vi "Assign Pixel to Wing Sector (FPGA).vi"(4 "End of Data?":bool, 6 "Valid Data?":bool, 7 "Pixel Intensity In":u8, 8 "Right Wing?":bool, 9 "Sector Parameters":T1, 10 "Pixel Y":u16, 11 "Pixel X":u16) -> (0 "Y Pixel Out":u16, 1 "Pixel Intensity Out":u8, 2 "sector #":u8, 3 "output valid":bool, 5 "X Pixel Out":u16)   [LabVIEW 2013]
uses:
  Sector Parameter Cluster.ctl
  <vilib>/rvi/FXPMathLib/FxpRectToPolar/XNode/nifxpmath_RectToPolar.xnode
  <vilib>/rvi/FXPMathLib/FxpSub/XNode/nifxpmath_Sub.xnode
  <vilib>/rvi/FXPMathLib/sim/FxpSim.dll
  <vilib>/rvi/FXPMathLib/FxpAdd/XNode/nifxpmath_Add.xnode
  <vilib>/rvi/FXPMathLib/FxpDiv/XNode/nifxpmath_Div.xnode
  <vilib>/rvi/FXPMathLib/FxpRectToPolar/simVIs/DllFxpRectToPolarTemp_sub.vi
  <vilib>/rvi/FXPMathLib/FxpRectToPolar/subVIs/nifxpmath_RectToPolar_SimConfig.ctl
  <vilib>/ptbypt/NI_PtbyPt.lvlib
  <vilib>/rvi/FXPMathLib/FxpDiv/simVIs/DllFxpDivTemp_sub.vi
  <vilib>/rvi/FXPMathLib/FxpDiv/subVIs/nifxpmath_Div_SimConfig.ctl
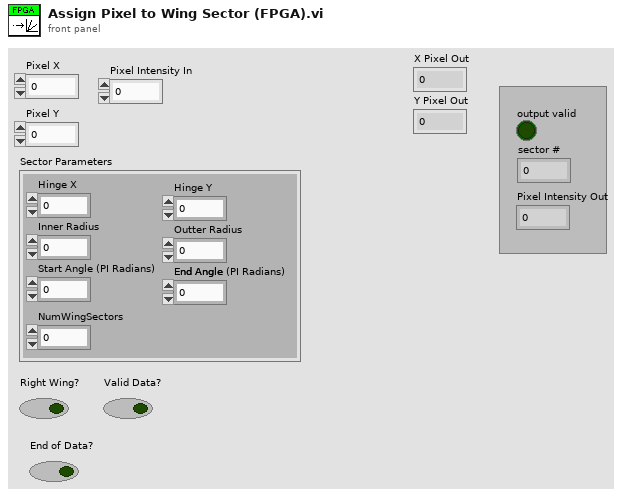
[diagram p1: front panel]
types:
  T1 = typedef "Sector Parameter Cluster.ctl" = cluster{"Start Angle":fxp<+/-,17,2>, "End Angle":fxp<+/-,17,2>, "Inner Radius":u16, "Outter Radius":u16, "Hinge X":u16, "Hinge Y":u16, "NumWingSectors":u8}
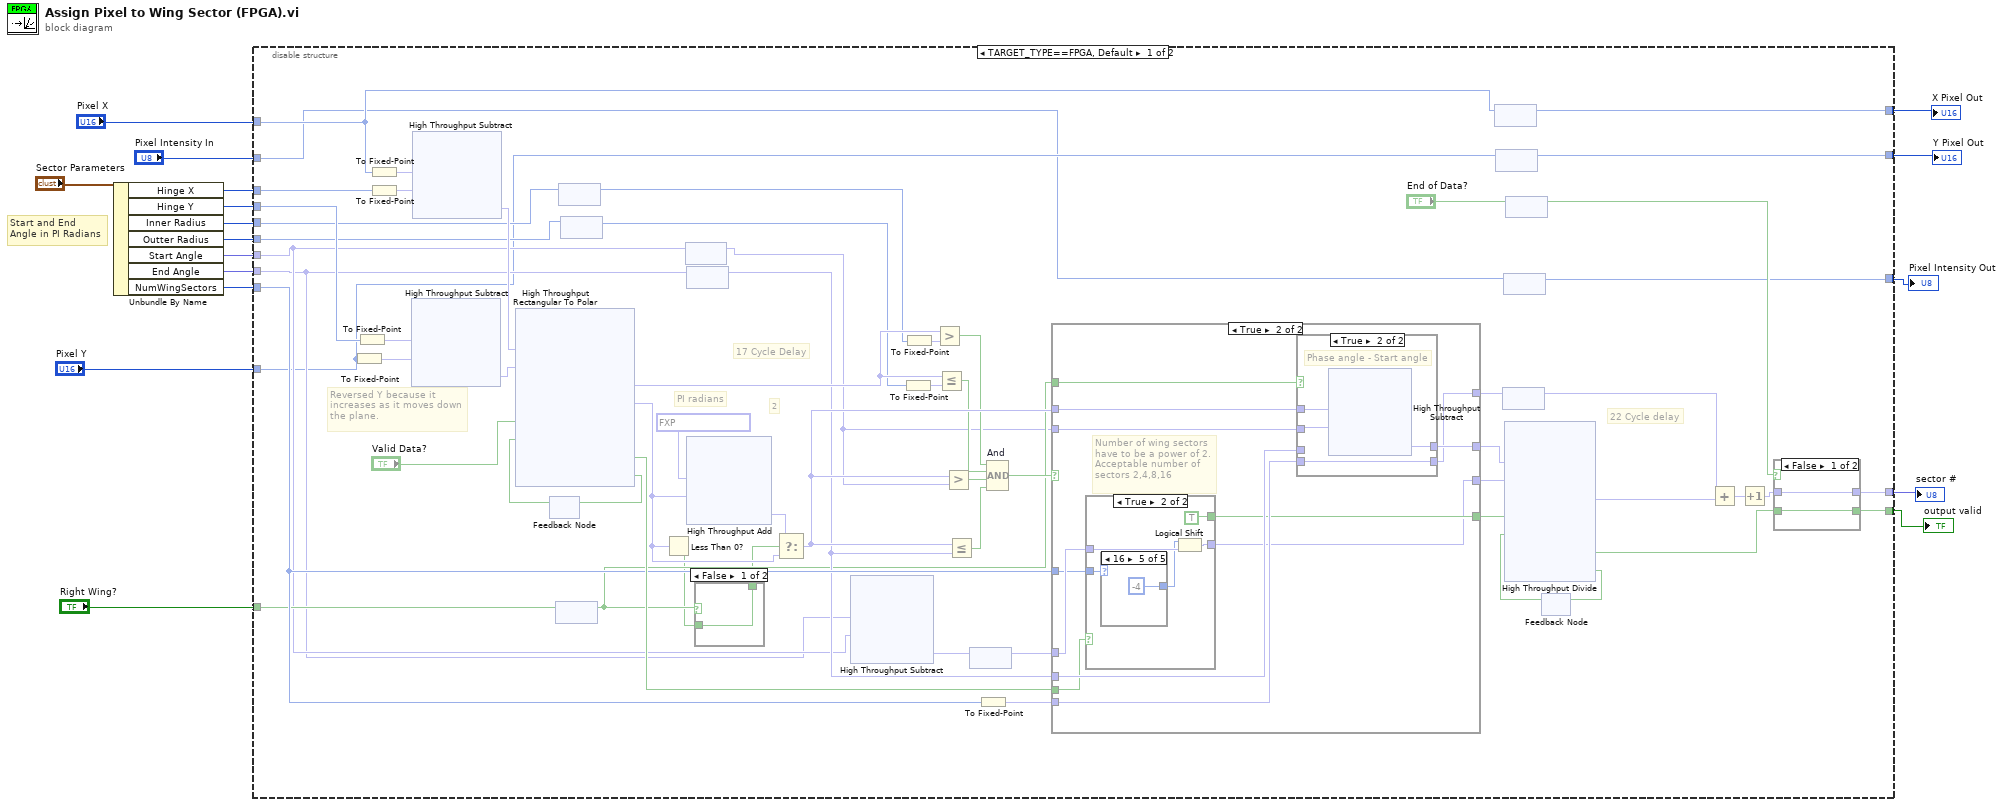
[diagram p0: block diagram]
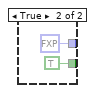
[diagram p2: hidden frame]
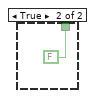
[diagram p3: hidden frame]
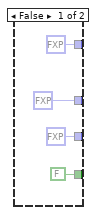
[diagram p4: hidden frame]
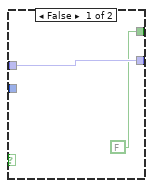
[diagram p5: hidden frame]
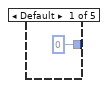
[diagram p6: hidden frame]
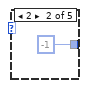
[diagram p7: hidden frame]
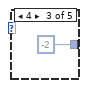
[diagram p8: hidden frame]
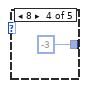
[diagram p9: hidden frame]
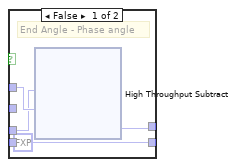
[diagram p10: hidden frame]
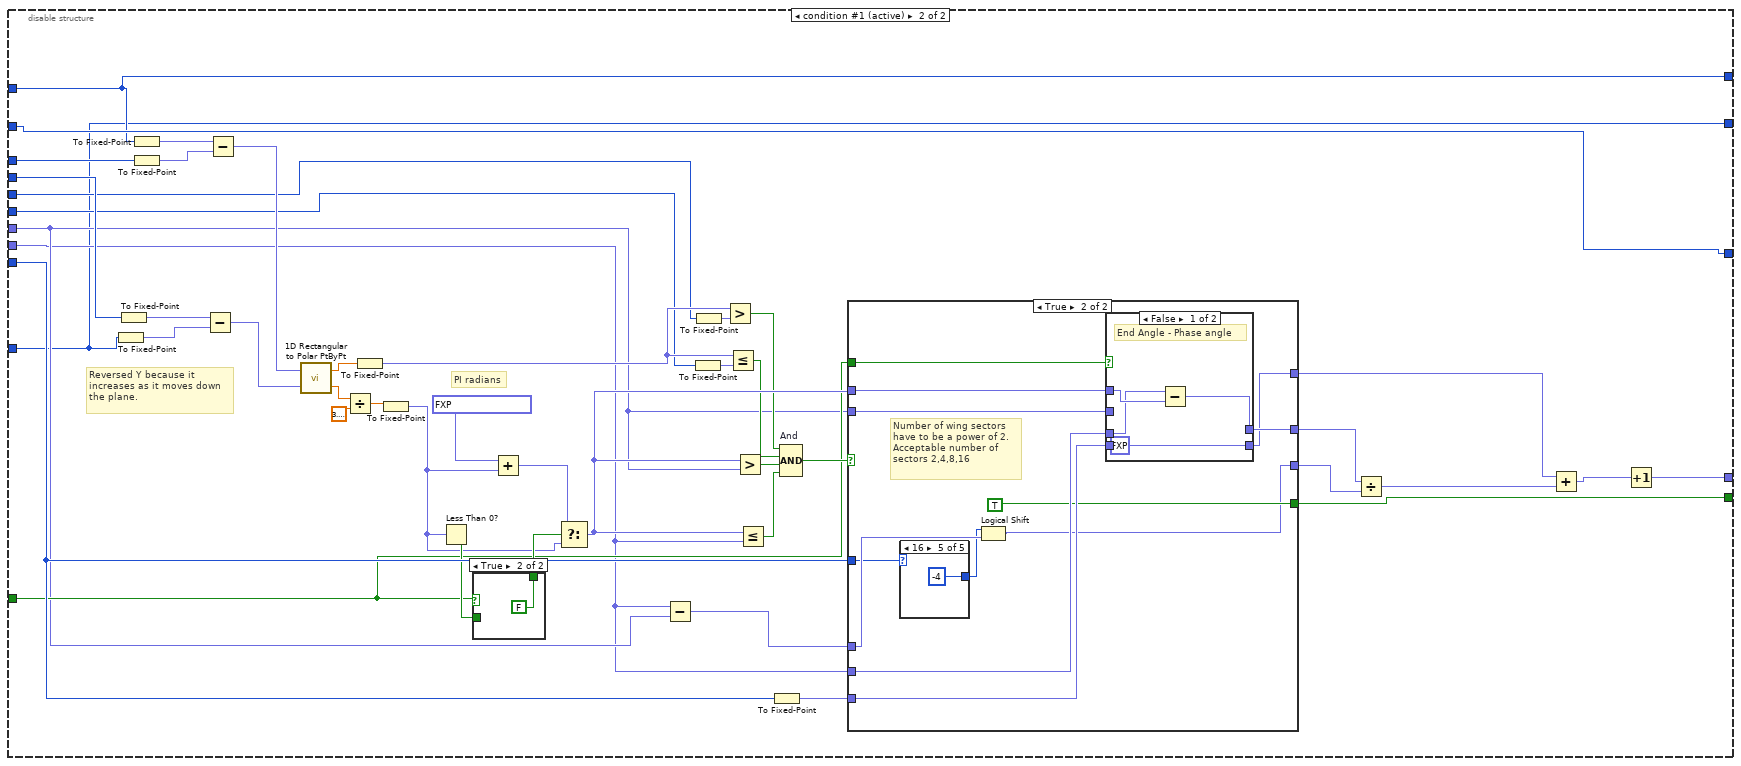
[diagram p11: hidden frame]
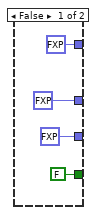
[diagram p13: hidden frame]
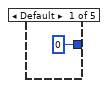
[diagram p14: hidden frame]
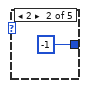
[diagram p15: hidden frame]
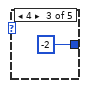
[diagram p16: hidden frame]
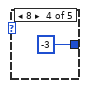
[diagram p17: hidden frame]
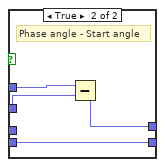
[diagram p18: hidden frame]
diagram:
  # "Start and End\nAngle in PI Radians"
  n1 = Unbundle By Name("Sector Parameters") -> ("Hinge X"=w15:u16, "Hinge Y"=w17:u16, "Inner Radius"=w13:u16, "Outter Radius"=w12:u16, "Start Angle"=w10:fxp<+/-,17,2>, "End Angle"=w9:fxp<+/-,17,2>, "NumWingSectors"=w16:u8)
  n2 = disable-structure shown="TARGET_TYPE==FPGA, Default" {
    disable-tunnel: w17 -> [w64 w222]
    disable-tunnel: w16 -> [w50 w214]
    disable-tunnel: w15 -> [w49 w213]
    disable-tunnel: w13 -> [w48 w202]
    disable-tunnel: w12 -> [w46 w201]
    disable-tunnel: "Right Wing?" -> [w40 w203]
    disable-tunnel: w10 -> [w37 w200]
    disable-tunnel: w9 -> [w35 w199]
    disable-tunnel: [w29 w190] -> w8
    disable-tunnel: [w27 w194] -> w7
    disable-tunnel: "Pixel X" -> [w25 w196]
    disable-tunnel: "Pixel Y" -> [w24 w195]
    disable-tunnel: [w23 w196] -> w4
    disable-tunnel: [w22 w195] -> w3
    disable-tunnel: [w21 w197] -> w2
    disable-tunnel: "Pixel Intensity In" -> [w20 w197]
    frame condition #0 {
      # "17 Cycle Delay"
      # "Reversed Y because it\nincreases as it moves down\nthe plane."
      # "PI radians"
      # "22 Cycle delay"
      # "2"
      n3 = To Fixed-Point(number=w24) -> (fixed-point=w54:fxp<+,11,11>)  [unwired: 1 in]
      n4 = To Fixed-Point(number=w64) -> (fixed-point=w55:fxp<+,11,11>)  [unwired: 1 in]
      n5 = To Fixed-Point(number=w25) -> (fixed-point=w53:fxp<+,11,11>)  [unwired: 1 in]
      n6 = To Fixed-Point(number=w49) -> (fixed-point=w52:fxp<+,11,11>)  [unwired: 1 in]
      n7 = xnode "High Throughput Subtract"("x"=w55, "y"=w54) -> ("x-y"=w63:fxp<+/-,12,12>)
      n8 = xnode "High Throughput Subtract"("x"=w53, "y"=w52) -> ("x-y"=w62:fxp<+/-,12,12>)
      n9 = feedback #1() -> (w69:bool)  [unwired: 1 in]
      n10 = xnode "High Throughput Rectangular To Polar"("x"=w62, "y"=w63, "input valid"="Valid Data?", "ready for output (T)"=w69) -> ("magnitude"=w77:fxp<+,12,12>, "phase (pi)"=w74:fxp<+/-,16,2>, "output valid"=w51:bool, "ready for input"=w70:bool)
      n11 = feedback-in #1(w70) -> ()
      n12 = feedback #2() -> (w43:bool)  [unwired: 1 in]
      n13 = feedback-in #2(w40) -> ()
      n14 = feedback #3() -> (w47:u16)  [unwired: 1 in]
      n15 = feedback-in #3(w48) -> ()
      n16 = feedback #4() -> (w45:u16)  [unwired: 1 in]
      n17 = feedback-in #4(w46) -> ()
      n18 = Less Than 0?(x=w74) -> (x < 0?=w41:bool)
      n19 = feedback #5() -> (w36:fxp<+/-,17,2>)  [unwired: 1 in]
      n20 = feedback-in #5(w37) -> ()
      n21 = xnode ("High Throughput Add")("x"=fxp<+/-,16,2> 1.99993896484375 ("y"), "y"=w74) -> ("x+y"=w73:fxp<+/-,17,3>)
      n22 = feedback #6() -> (w44:fxp<+/-,17,2>)  [unwired: 1 in]
      n23 = feedback-in #6(w35) -> ()
      n24 = case shown="False" w43 {
        tunnel: [w83 FALSE ("s")] -> w42
        tunnel: w41 -> [w83 _]
        frame False {
        }
        frame True {
        }
      }
      n25 = Select(t=w73, s=w42, f=w74) -> (s? t:f=w71:fxp<+/-,17,3>)
      n26 = xnode ("High Throughput Subtract")("x"=w35, "y"=w37) -> ("x-y"=w34:fxp<+/-,18,3>)
      n27 = To Fixed-Point(number=w45) -> (fixed-point=w76:fxp<+,16,16>)  [unwired: 1 in]
      n28 = To Fixed-Point(number=w47) -> (fixed-point=w78:fxp<+,16,16>)  [unwired: 1 in]
      n29 = Greater?(x=w77, y=w78) -> (0:w68:bool)
      n30 = Less Or Equal?(x=w77, y=w76) -> (x <= y?=w67:bool)
      n31 = Greater?(x=w71, y=w36) -> (0:w66:bool)
      n32 = Less Or Equal?(x=w71, y=w44) -> (x <= y?=w65:bool)
      n33 = feedback #7() -> (w33:fxp<+/-,18,3>)  [unwired: 1 in]
      n34 = feedback-in #7(w34) -> ()
      n35 = To Fixed-Point(number=w50) -> (fixed-point=w39:fxp<+,8,8>)  [unwired: 1 in]
      n36 = Compound Arithmetic op=AND "And"(w68, w67, w66, w65) -> (w75:bool)
      n37 = case shown="True" w75 {
        tunnel: w71 -> [_ w129]
        tunnel: w36 -> [_ w128]
        tunnel: [fxp<+/-,18,3> 0.0 ("x-y") w119] -> w59
        tunnel: w44 -> [_ w126]
        tunnel: w39 -> [_ w127]
        tunnel: [fxp<+/-,20,5> 0.0 ("x-y") w125] -> w60
        tunnel: [FALSE ("output valid") w120] -> w58
        tunnel: [fxp<+,8,8> 0.0 w124] -> w56
        tunnel: w33 -> [_ w123]
        tunnel: w51 -> [_ w122]
        tunnel: w50 -> [_ w121]
        tunnel: w43 -> [_ w118]
        frame False {
        }
        frame True {
          # "Number of wing sectors\nhave to be a power of 2.\nAcceptable number of\nsectors 2,4,8,16"
          n38 = case shown="True" w122 {
            tunnel: w121 -> [_ w136]
            tunnel: w123 -> [w131 w135]
            tunnel: [w131 w133] -> w119
            tunnel: [FALSE ("output valid") TRUE ("output valid")] -> w120
            frame False {
            }
            frame True {
              n39 = case shown="16" w136 {
                tunnel: [i16 0 ("y") i16 -1 ("y") i16 -2 ("y") i16 -3 ("y") i16 -4 ("y")] -> w134
                frame Default {
                }
                frame 2 {
                }
                frame 4 {
                }
                frame 8 {
                }
                frame 16 {
                }
              }
              n40 = Logical Shift(y=w134, x=w135) -> (x << y=w133:fxp<+/-,18,3>)
            }
          }
          n41 = case shown="True" w118 {
            tunnel: w129 -> [w144 w149]
            tunnel: w128 -> [_ w148]
            tunnel: [w145 w147] -> w125
            tunnel: w127 -> [_ w146]
            tunnel: [fxp<+,8,8> 0.0 w146] -> w124
            tunnel: w126 -> [w143 _]
            frame False {
              # "End Angle - Phase angle"
              n42 = xnode "High Throughput Subtract"("x"=w143, "y"=w144) -> ("x-y"=w145:fxp<+/-,19,4>)
            }
            frame True {
              # "Phase angle - Start angle"
              n43 = xnode ("High Throughput Subtract")("x"=w149, "y"=w148) -> ("x-y"=w147:fxp<+/-,19,4>)
            }
          }
        }
      }
      n44 = feedback #8() -> (w23:u16)  [unwired: 1 in]
      n45 = feedback-in #8(w25) -> ()
      n46 = feedback #9() -> (w22:u16)  [unwired: 1 in]
      n47 = feedback-in #9(w24) -> ()
      n48 = feedback #10() -> (w38:fxp<+,8,8>)  [unwired: 1 in]
      n49 = feedback-in #10(w56) -> ()
      n50 = feedback #11() -> (w21:u8)  [unwired: 1 in]
      n51 = feedback-in #11(w20) -> ()
      n52 = feedback #12() -> (w30:bool)  [unwired: 1 in]
      n53 = feedback-in #12("End of Data?") -> ()
      n54 = feedback #13() -> (w57:bool)  [unwired: 1 in]
      n55 = xnode "High Throughput Divide"("x"=w60, "y"=w59, "input valid"=w58, "ready for output (T)"=w57) -> ("x/y"=w19:fxp<+/-,20,20>, "output valid"=w26:bool, "ready for input"=w61:bool)
      n56 = feedback-in #13(w61) -> ()
      n57 = Add(x=w38, y=w19) -> (x+y=w28:fxp<+/-,21,21>)
      n58 = Increment(x=w28) -> (x+1=w18:fxp<+/-,21,21>)
      n59 = case shown="False" w30 {
        tunnel: [w80 fxp<+/-,17,17> 0.0] -> w29
        tunnel: w18 -> [w80 _]
        tunnel: [w79 TRUE ("output valid")] -> w27
        tunnel: w26 -> [w79 _]
        frame False {
        }
        frame True {
        }
      }
    }
    frame condition #1 (active) {
      # "Reversed Y because it\nincreases as it moves down\nthe plane."
      # "PI radians"
      n60 = To Fixed-Point(number=w195) -> (fixed-point=w217:fxp<+,11,11>)  [unwired: 1 in]
      n61 = To Fixed-Point(number=w222) -> (fixed-point=w218:fxp<+,11,11>)  [unwired: 1 in]
      n62 = To Fixed-Point(number=w196) -> (fixed-point=w216:fxp<+,11,11>)  [unwired: 1 in]
      n63 = To Fixed-Point(number=w213) -> (fixed-point=w215:fxp<+,11,11>)  [unwired: 1 in]
      n64 = Subtract(x=w218, y=w217) -> (x-y=w221:fxp<+/-,12,12>)
      n65 = Subtract(x=w216, y=w215) -> (x-y=w220:fxp<+/-,12,12>)
      n66 = call <vilib>:"1D Rectangular to Polar PtByPt.vi"("y"=w221, "x"=w220) -> ("phase"=w207:dbl, "magnitude"=w209:dbl)
      n67 = Divide(x=w207, y=3.141592653589793) -> (x/y=w205:dbl)
      n68 = To Fixed-Point(number=w209) -> (fixed-point=w208:fxp<+,12,12>)  [unwired: 1 in]
      n69 = To Fixed-Point(number=w205) -> (fixed-point=w204:fxp<+/-,16,2>)  [unwired: 1 in]
      n70 = Less Than 0?(x=w204) -> (x < 0?=w211:bool)
      n71 = case shown="True" w203 {
        tunnel: [w233 FALSE ("s")] -> w212
        tunnel: w211 -> [w233 _]
        frame False {
        }
        frame True {
        }
      }
      n72 = Add(x=fxp<+/-,16,2> 1.99993896484375 ("y"), y=w204) -> (x+y=w229:fxp<+/-,17,3>)
      n73 = Select(t=w229, s=w212, f=w204) -> (s? t:f=w227:fxp<+/-,17,3>)
      n74 = Subtract(x=w199, y=w200) -> (x-y=w198:fxp<+/-,18,3>)
      n75 = To Fixed-Point(number=w201) -> (fixed-point=w231:fxp<+,16,16>)  [unwired: 1 in]
      n76 = To Fixed-Point(number=w202) -> (fixed-point=w232:fxp<+,16,16>)  [unwired: 1 in]
      n77 = Greater?(x=w208, y=w232) -> (0:w226:bool)
      n78 = Less Or Equal?(x=w208, y=w231) -> (x <= y?=w225:bool)
      n79 = Greater?(x=w227, y=w200) -> (0:w224:bool)
      n80 = Less Or Equal?(x=w227, y=w199) -> (x <= y?=w223:bool)
      n81 = To Fixed-Point(number=w214) -> (fixed-point=w210:fxp<+,8,8>)  [unwired: 1 in]
      n82 = Compound Arithmetic op=AND "And"(w226, w225, w224, w223) -> (w230:bool)
      n83 = case shown="True" w230 {
        tunnel: w227 -> [_ w250]
        tunnel: w200 -> [_ w249]
        tunnel: [fxp<+/-,18,3> 0.0 ("x-y") w241] -> w192
        tunnel: w199 -> [_ w247]
        tunnel: w210 -> [_ w248]
        tunnel: [fxp<+/-,20,5> 0.0 ("x-y") w246] -> w219
        tunnel: [FALSE ("output valid") TRUE ("output valid")] -> w194
        tunnel: [fxp<+,8,8> 0.0 w245] -> w193
        tunnel: w198 -> [_ w244]
        tunnel: w214 -> [_ w243]
        tunnel: w203 -> [_ w240]
        frame False {
        }
        frame True {
          # "Number of wing sectors\nhave to be a power of 2.\nAcceptable number of\nsectors 2,4,8,16"
          n84 = case shown="16" w243 {
            tunnel: [i16 0 ("y") i16 -1 ("y") i16 -2 ("y") i16 -3 ("y") i16 -4 ("y")] -> w239
            frame Default {
            }
            frame 2 {
            }
            frame 4 {
            }
            frame 8 {
            }
            frame 16 {
            }
          }
          n85 = Logical Shift(y=w239, x=w244) -> (x << y=w241:fxp<+/-,18,3>)
          n86 = case shown="False" w240 {
            tunnel: w250 -> [w258 w263]
            tunnel: w249 -> [_ w262]
            tunnel: [w259 w261] -> w246
            tunnel: w248 -> [_ w260]
            tunnel: [fxp<+,8,8> 0.0 w260] -> w245
            tunnel: w247 -> [w257 _]
            frame False {
              # "End Angle - Phase angle"
              n87 = Subtract(x=w257, y=w258) -> (x-y=w259:fxp<+/-,19,4>)
            }
            frame True {
              # "Phase angle - Start angle"
              n88 = Subtract(x=w263, y=w262) -> (x-y=w261:fxp<+/-,19,4>)
            }
          }
        }
      }
      n89 = Divide(x=w219, y=w192) -> (x/y=w189:fxp<+/-,20,20>)
      n90 = Add(x=w193, y=w189) -> (x+y=w191:fxp<+/-,21,21>)
      n91 = Increment(x=w191) -> (x+1=w190:fxp<+/-,21,21>)
    }
  }
  "output valid" <- w7
  "sector #" <- w8
  "X Pixel Out" <- w4
  "Y Pixel Out" <- w3
  "Pixel Intensity Out" <- w2
